vi "ProcessFolder.vi"(11 "Path":path) -> (3 "Array":cluster{"Source path":path, "Dest Path":path}[](array[cluster]))   [LabVIEW 2014]
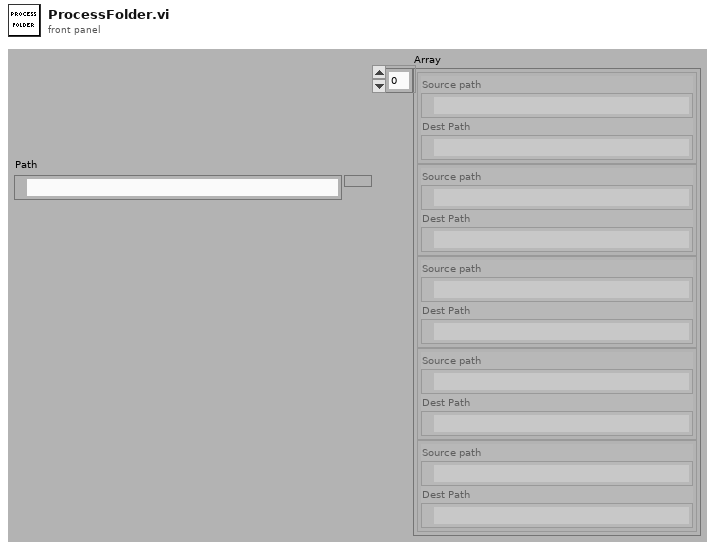
[diagram p1: front panel]
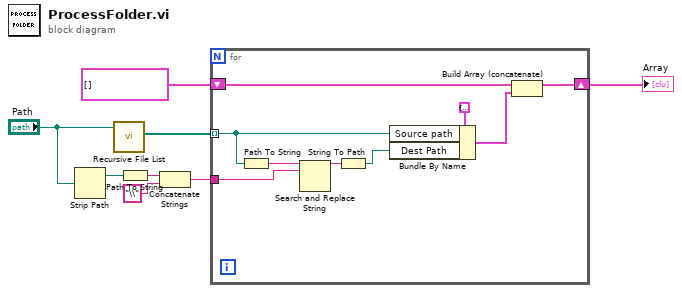
[diagram p0: block diagram]
diagram:
  n1 = Strip Path(path="Path") -> (stripped path=w1:path)  [unwired: 1 out]
  n2 = call <vilib>:"Recursive File List.vi"("Folder Path"="Path") -> ("All Files in Dir"=w8:path[])  [unwired: 6 in, 4 out]
  n3 = Path To String(path=w1) -> (string=w7:string)
  n4 = Concatenate Strings(w7, "\\" ("string")) -> (w5:string)
  n5 = for {
    tunnel: w8 -> [w14] mode=indexing
    tunnel: w5 -> [w16]
    shift-right: [w9] -> w3
    shift-left: cluster{"Source path":path, "Dest Path":path}[] [] -> [w11]
    n6 = Path To String(path=w14) -> (string=w17:string)
    n7 = Search and Replace String(input string=w17, search string=w16) -> (result string=w13:string)  [unwired: 6 in, 3 out]
    n8 = String To Path(string=w13) -> (path=w12:path)
    n9 = Bundle By Name(cluster=cluster{"Source path":path, "Dest Path":path} {"Source path"=path "", "Dest Path"=path ""}, "Source path"=w14, "Dest Path"=w12) -> (w10:cluster{"Source path":path, "Dest Path":path})
    n10 = Build Array (concatenate)(w11, w10) -> (w9:cluster{"Source path":path, "Dest Path":path}[])
  }
  "Array" <- w3
